vi "Hashes Example.vi"(9 "pipelining enabled?":bool=TRUE, 10 "# of keys to test":i32=500) -> (0 "error out":errorcluster, 1 "set = get?":bool, 2 "# of fields added":i64, 4 "execution time (ms/key)":dbl, 5 "KEY":string)   [LabVIEW 2023, in "Redis Client Examples.lvlib"]
uses:
  Redis Client Examples.lvlib
  <vilib>/numeric/Random Number (Range) I64.vi
  <vilib>/numeric/sub_Random U32.vi
  Redis Client for LabVIEW/Redis Pipelining TCP Client/Redis Pipelining TCP Client.lvclass
  home/enrico/Eran/LAST/Redis-Labview/Redis-Client-for-LabVIEW/Redis Client for LabVIEW/Redis Client/Redis Client.lvclass
  Redis Client for LabVIEW/Redis Pipelining TCP Client/impl/set pipelining.vi
  lib/RESP3-for-LabVIEW/RESP3/high-level/RESP3 Get String.vi
  Redis Client for LabVIEW/Redis Client/Redis Client.lvclass
  Redis Client for LabVIEW/Redis TCP Client/Redis TCP Client.lvclass
  lib/RESP3-for-LabVIEW/RESP3/RESP3.lvlib
  home/enrico/Eran/LAST/Redis-Labview/Redis-Client-for-LabVIEW/Redis Client for LabVIEW/Redis TCP Client/Redis TCP Client.lvclass
  home/enrico/Eran/LAST/Redis-Labview/Redis-Client-for-LabVIEW/Redis Client for LabVIEW/Redis Pipelining TCP Client/Redis Pipelining TCP Client.lvclass
panel:
  out "ping response":variant
  out "server properties":variant
  out "client name":string
  out "client info":string
  out "client id":i64 format="%.0x"
  out "Pipeline: RESP3 Values":variant[](array[variant])
  out "all keys found?":bool
  out "iter#":i32=49
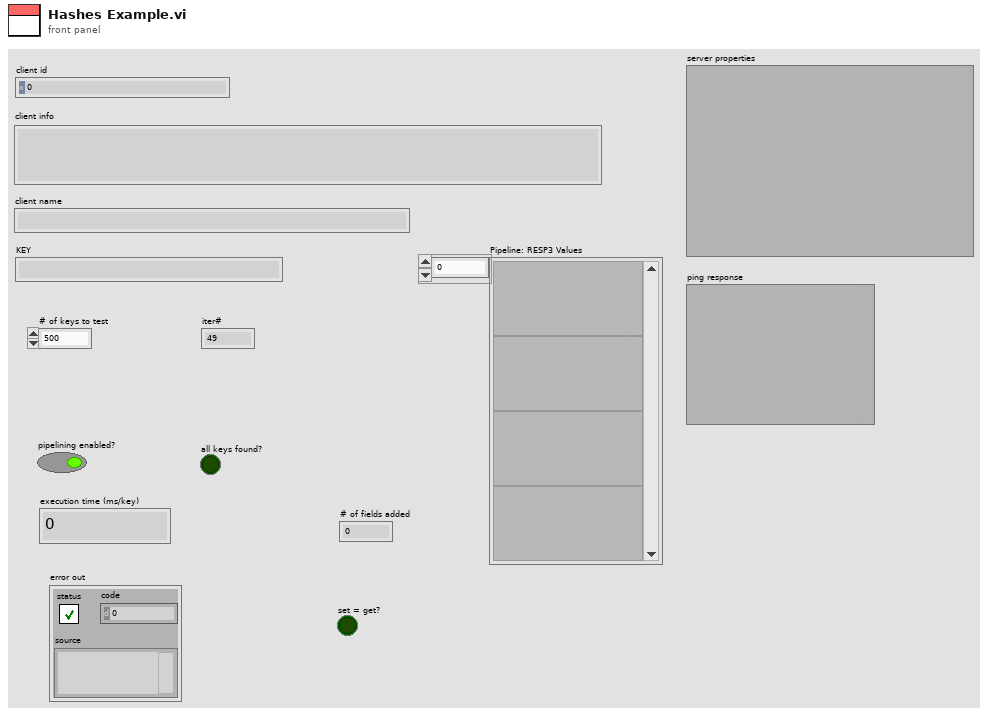
[diagram p1: front panel]
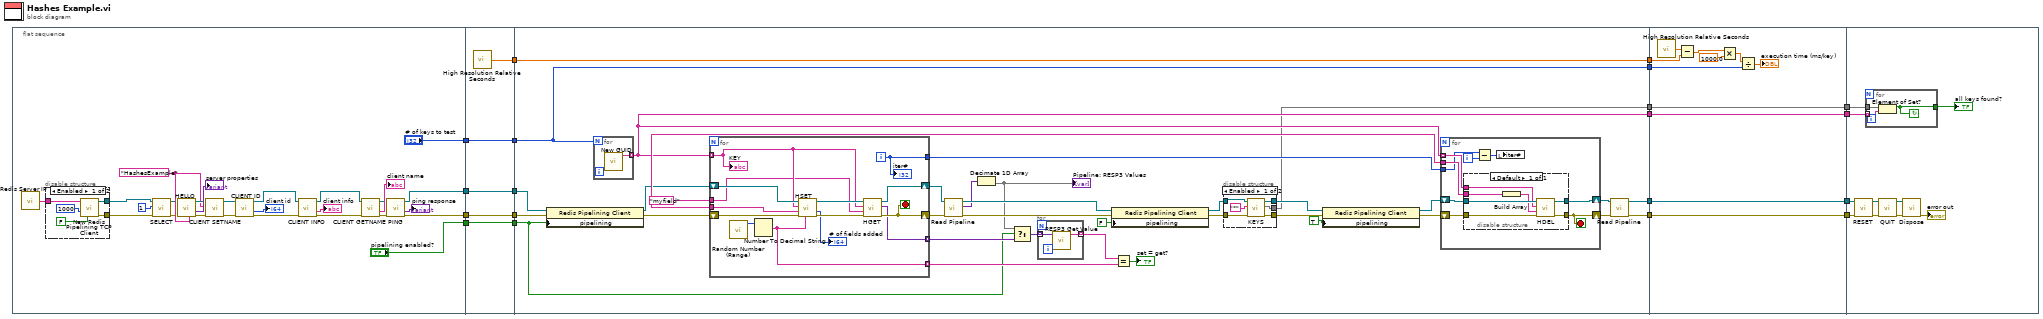
[diagram p0: block diagram]
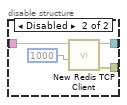
[diagram p2: hidden frame]
diagram:
  n1 = flat-sequence {
    tunnel: [w29] -> w15
    tunnel: [w30] -> w13
    tunnel: ["# of keys to test"] -> w7
    tunnel: ["pipelining enabled?"] -> w5
    tunnel: [w59] -> w18
    tunnel: [w58] -> w16
    tunnel: w15 -> [w58]
    tunnel: [w57] -> w14
    tunnel: w13 -> [w57]
    tunnel: [w56] -> w8
    tunnel: w7 -> [w56]
    tunnel: [w55] -> w6
    tunnel: w5 -> [w55]
    tunnel: [w91] -> w19
    tunnel: w18 -> [w91]
    tunnel: [w66] -> w17
    tunnel: w16 -> [w73]
    tunnel: w14 -> [w72]
    tunnel: [w71] -> w11
    tunnel: [w70] -> w9
    tunnel: w8 -> [w66]
    tunnel: w6 -> [w62]
    tunnel: [w61] -> w3
    tunnel: [w60] -> w1
    tunnel: w19 -> [w144]
    tunnel: w17 -> [w139]
    tunnel: [w138] -> w12
    tunnel: w11 -> [w138]
    tunnel: [w137] -> w10
    tunnel: w9 -> [w137]
    tunnel: [w136] -> w4
    tunnel: w3 -> [w136]
    tunnel: [w135] -> w2
    tunnel: w1 -> [w135]
    tunnel: w12 -> [w152]
    tunnel: w10 -> [w153]
    tunnel: w4 -> [w147]
    tunnel: w2 -> [w146]
    frame #0 {
      w33 = "HashesExample" ("client name")
      n2 = call "Redis Server IP.vi"() -> ("server IP"=w34:string)
      n3 = disable-structure shown="Enabled" {
        disable-tunnel: w34 -> [w50 w54]
        disable-tunnel: [w49 w52] -> w25
        disable-tunnel: [w48 w51] -> w26
        frame Enabled {
          n4 = call "New Redis Pipelining TCP Client.vi"("pipelining enabled?"=FALSE, "timeout ms (25000)"=1000, "address"=w50) -> ("error out"=w49:errorcluster, "Redis Pipelining TCP Client out"=w48:refnum<class "Redis Pipelining TCP Client.lvclass">)  [unwired: 7 in]
        }
        frame Disabled {
          n5 = call "New Redis TCP Client.vi"("timeout ms (25000)"=1000, "address"=w54) -> ("error out"=w52:errorcluster, "Redis TCP Client out"=w51:refnum<class "Redis TCP Client.lvclass">)  [unwired: 8 in]
        }
      }
      n6 = call "SELECT.vi"("error in (no error)"=w25, "index"=i64 1, "Redis Client in"=w26) -> ("error out"=w23:errorcluster, "Redis Client out"=w24:refnum<class "Redis Pipelining TCP Client.lvclass">)  [unwired: 6 in, 1 out]
      n7 = call "HELLO.vi"("client name"=w33, "error in (no error)"=w23, "Redis Client in"=w24) -> ("error out"=w43:errorcluster, "server properties"=→"server properties":variant, "Redis Client out"=w44:refnum<class "Redis Pipelining TCP Client.lvclass">)  [unwired: 6 in]
      n8 = call "CLIENT SETNAME.vi"("error in (no error)"=w43, "client name"=w33, "Redis Client in"=w44) -> ("error out"=w42:errorcluster, "Redis Client out"=w41:refnum<class "Redis Pipelining TCP Client.lvclass">)  [unwired: 6 in, 1 out]
      n9 = call "CLIENT ID.vi"("error in (no error)"=w42, "Redis Client in"=w41) -> ("error out"=w37:errorcluster, "client id"=→"client id":i64, "Redis Client out"=w36:refnum<class "Redis Pipelining TCP Client.lvclass">)  [unwired: 7 in]
      n10 = call "CLIENT INFO.vi"("error in (no error)"=w37, "Redis Client in"=w36) -> ("error out"=w40:errorcluster, "client info"=→"client info":string, "Redis Client out"=w39:refnum<class "Redis Pipelining TCP Client.lvclass">)  [unwired: 7 in]
      n11 = call "CLIENT GETNAME.vi"("error in (no error)"=w40, "Redis Client in"=w39) -> ("error out"=w28:errorcluster, "client name"=→"client name":string, "Redis Client out"=w31:refnum<class "Redis Pipelining TCP Client.lvclass">)  [unwired: 7 in]
      n12 = call "PING.vi"("error in (no error)"=w28, "Redis Client in"=w31) -> ("error out"=w29:errorcluster, "response"=→"ping response":variant, "Redis Client out"=w30:refnum<class "Redis Pipelining TCP Client.lvclass">)  [unwired: 7 in]
    }
    frame #1 {
      n13 = call <vilib>:"High Resolution Relative Seconds.vi"() -> ("relative seconds"=w59:dbl)
    }
    frame #2 {
      w93 = "myfield" ("field")
      n14 = property class="Redis Pipelining Client"(reference=w72, error in=w73, "pipelining"=w62) -> (reference out=w75:refnum<class "Redis Pipelining TCP Client.lvclass">, error out=w74:errorcluster)
      n15 = for {
        N: w66 -> [_]
        tunnel: [w120] -> w61 mode=indexing
        n16 = call "New GUID.vi"() -> ("ToString"=w120:string)  [unwired: 11 in]
      }
      n17 = for {
        shift-right: [w129] -> w90
        shift-left: w75 -> [w134]
        shift-right: [w125] -> w89
        shift-left: w74 -> [w133]
        tunnel: w61 -> [w130] mode=indexing
        tunnel: w93 -> [w128]
        tunnel: w93 -> [w127]
        tunnel: [w126] -> w92
        tunnel: [w123] -> w69 mode=indexing
        tunnel: [w121] -> w64 mode=indexing
        i -> [w126]
        stop <- w125 stop-if-true
        n18 = call-poly <vilib>:"Random Number (Range).vi"() -> ("number"=w124:i64)  [unwired: 11 in]
        n19 = Number To Decimal String(number=w124) -> (decimal integer string=w123:string)  [unwired: 1 in]
        n20 = call "HSET.vi"("string value"=w123, "error in (no error)"=w133, "field"=w127, "key"=w130, "Redis Client in"=w134) -> ("error out"=w131:errorcluster, "# of fields added"=→"# of fields added":i64, "Redis Client out"=w132:refnum<class "Redis Pipelining TCP Client.lvclass">)  [unwired: 4 in]
        n21 = call "HGET.vi"("error in (no error)"=w131, "field"=w128, "key"=w130, "Redis Client in"=w132) -> ("error out"=w125:errorcluster, "RESP3 Value"=w121:variant, "Redis Client out"=w129:refnum<class "Redis Pipelining TCP Client.lvclass">)  [unwired: 4 in, 1 out]
        "KEY" <- w130
        "iter#" <- w126
      }
      n22 = call "Read Pipeline.vi"("error in (no error)"=w89, "Redis Pipelining Client in"=w90) -> ("error out"=w81:errorcluster, "RESP3 Values"=w76:variant[], "Redis Pipelining Client out"=w88:refnum<class "Redis Pipelining TCP Client.lvclass">)  [unwired: 6 in, 1 out]
      n23 = Decimate 1D Array(w76) -> (w63:variant[])  [unwired: 1 out]
      "Pipeline: RESP3 Values" <- w63
      n24 = Select(t=w63, s=w62, f=w64) -> (s? t:f=w65:variant[])
      n25 = for {
        tunnel: w65 -> [w95] mode=indexing
        tunnel: [w94] -> w67 mode=indexing
        n26 = call-poly "RESP3 Get Value.vi"("RESP3 Value in"=w95) -> ("String out"=w94:string)  [unwired: 7 in, 3 out]
      }
      n27 = property class="Redis Pipelining Client"(reference=w88, error in=w81, "pipelining"=FALSE) -> (reference out=w84:refnum<class "Redis Pipelining TCP Client.lvclass">, error out=w80:errorcluster)
      n28 = Equal?(x=w67, y=w69) -> (x = y?=→"set = get?":bool)
      n29 = disable-structure shown="Enabled" {
        disable-tunnel: [w100 _] -> w60
        disable-tunnel: [w99 w103] -> w85
        disable-tunnel: w84 -> [w98 w103]
        disable-tunnel: [w97 w102] -> w82
        disable-tunnel: w80 -> [w96 w102]
        frame Enabled {
          n30 = call "KEYS.vi"("error in (no error)"=w96, "pattern"="*", "Redis Client in"=w98) -> ("error out"=w97:errorcluster, "keys"=w100:set{string}, "Redis Client out"=w99:refnum<class "Redis Pipelining TCP Client.lvclass">)  [unwired: 6 in]
        }
        frame Disabled {
        }
      }
      n31 = property class="Redis Pipelining Client"(reference=w85, error in=w82, "pipelining"=TRUE) -> (reference out=w83:refnum<class "Redis Pipelining TCP Client.lvclass">, error out=w79:errorcluster)
      n32 = for {
        shift-right: [w112] -> w87
        shift-left: w83 -> [w108]
        shift-right: [w104] -> w86
        shift-left: w79 -> [w111]
        tunnel: w61 -> [w110] mode=indexing
        tunnel: w93 -> [w109]
        tunnel: w92 -> [w106]
        i -> [w107]
        stop <- w104 stop-if-true
        n33 = disable-structure shown="Default" {
          disable-tunnel: w108 -> [w119]
          disable-tunnel: w111 -> [w118]
          disable-tunnel: [w117] -> w112
          disable-tunnel: [w116] -> w104
          disable-tunnel: w110 -> [w115]
          disable-tunnel: w109 -> [w114]
          frame Enabled {
            n34 = Build Array(w114) -> (w113:string[])
            n35 = call "HDEL.vi"("error in (no error)"=w118, "fields"=w113, "key"=w115, "Redis Client in"=w119) -> ("error out"=w116:errorcluster, "Redis Client out"=w117:refnum<class "Redis Pipelining TCP Client.lvclass">)  [unwired: 5 in, 1 out]
          }
        }
        n36 = Subtract(x=w106, y=w107) -> (x-y=w105:i32)
        n37 = local write "iter#"(w105) -> ()
      }
      n38 = call "Read Pipeline.vi"("error in (no error)"=w86, "Redis Pipelining Client in"=w87) -> ("error out"=w71:errorcluster, "Redis Pipelining Client out"=w70:refnum<class "Redis Pipelining TCP Client.lvclass">)  [unwired: 6 in, 2 out]
    }
    frame #3 {
      n39 = call <vilib>:"High Resolution Relative Seconds.vi"() -> ("relative seconds"=w145:dbl)
      n40 = Subtract(x=w145, y=w144) -> (x-y=w143:dbl)
      n41 = Multiply(x=w143, y=1000.0) -> (x*y=w141:dbl)
      n42 = Divide(x=w141, y=w139) -> (x/y=→"execution time (ms/key)":dbl)
    }
    frame #4 {
      n43 = call "RESET.vi"("error in (no error)"=w152, "Redis Client in"=w153) -> ("error out"=w151:errorcluster, "Redis Client out"=w154:refnum<class "Redis Pipelining TCP Client.lvclass">)  [unwired: 8 in]
      n44 = for {
        tunnel: w147 -> [w157] mode=indexing
        tunnel: w146 -> [w158]
        tunnel: [w156] -> w148
        stop <- w156 continue-if-true
        n45 = Element of Set?(10:w157, 11:w158) -> (3:w156:bool)
      }
      "all keys found?" <- w148
      n46 = call "QUIT.vi"("error in (no error)"=w151, "Redis Client in"=w154) -> ("error out"=w150:errorcluster, "Redis Client out"=w149:refnum<class "Redis Pipelining TCP Client.lvclass">)  [unwired: 8 in]
      n47 = call-dynamic "Dispose.vi"("error in (no error)"=w150, "Redis Pipelining TCP Client in"=w149) -> ("error out"=→"error out":errorcluster)  [unwired: 9 in]
    }
  }
